vi "Calculate Linear Calibration from measurements (1D).vi"(8 "error in (no error)":errorcluster, 10 "A*":dbl[](array[numeric]), 11 "A":dbl[](array[numeric])) -> (0 "error out":errorcluster, 3 "Linear Calibration 1D":T1)   [LabVIEW 2011, in "COSYLib.lvlib"]
uses:
  Linear Calibration 1D.ctl
  COSYLib.lvlib
  <vilib>/Analysis/NI_AALPro.lvlib
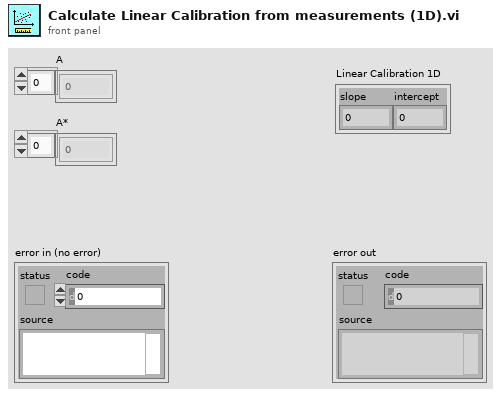
[diagram p1: front panel]
types:
  T1 = typedef "COSYLib.lvlib/Linear Calibration 1D.ctl" = cluster{"slope":dbl, "intercept":dbl}
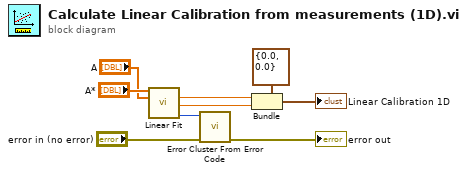
[diagram p0: block diagram]
diagram:
  n1 = call <vilib>:"Linear Fit.vi"("Y"="A*", "X"="A") -> ("slope"=w4:dbl, "intercept"=w3:dbl, "error"=w7:i32)  [unwired: 9 in, 2 out]
  n2 = call <vilib>:"Error Cluster From Error Code.vi"("error in (no error)"="error in (no error)", "error code (0)"=w7) -> ("error out"=→"error out":errorcluster)  [unwired: 7 in]
  n3 = Bundle(cluster=T1 {"slope"=0.0, "intercept"=0.0} ("Linear Calibration"), "slope"=w4, "intercept"=w3) -> (→"Linear Calibration 1D":T1)
